vi "save_file_from_netcat.vi"() -> ()   [LabVIEW 2018]
doc: "Demonstrates how to open a connection to an TCP server, read the data being sent, and display the data on a chart. This VI is designed to stop if the TCP connection is terminated."
panel:
  out "bytes received":i32
  out "data":string
  in  "Server Closed":string="The server VI closed the connection."
  in  "Stop":bool
  # "Overview: Demonstrates the use of the TCP functions to connect to a TCP server VI and receive data.\nInstructions:\n1. Ensure Simple TCP - Server.vi is already running.\n2. Run the VI.\n3. Click Stop to stop the VI. Note that if you stop the server VI, this VI will stop automatically."
  # "Send the file on sever using netcat:\nnc -T reliability 192.168.163.61 5901 < OpenSSH-Win64.zip"
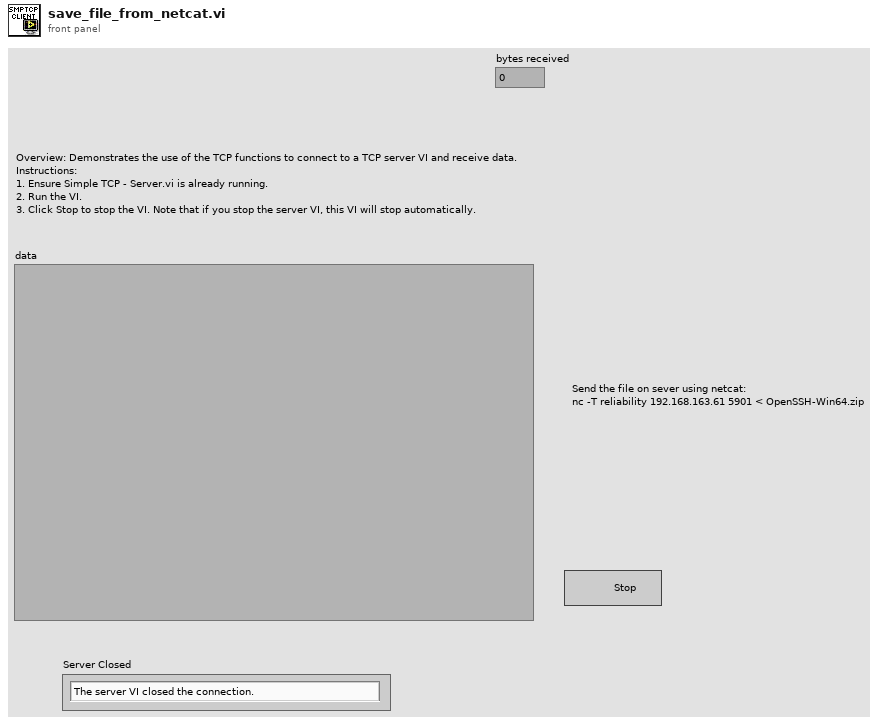
[diagram p1: front panel]
types:
  T1 = enum16{"open", "replace", "create", "open or create", "replace or create", "replace or create with confirmation"}
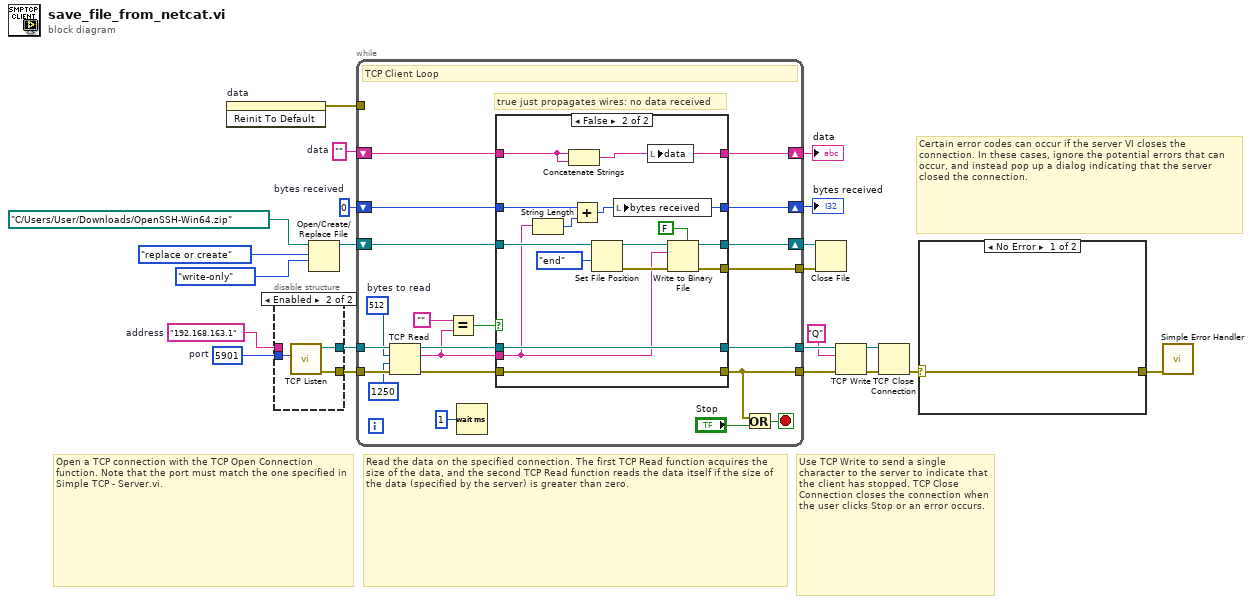
[diagram p0: block diagram]
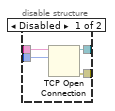
[diagram p2: hidden frame]
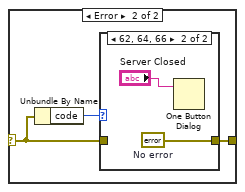
[diagram p3: hidden frame]
diagram:
  w2 = 0  # bytes received
  w11 = ""  # data
  w12 = u16 5901  # port
  w13 = "192.168.163.1"  # address
  # "Certain error codes can occur if the server VI closes the connection. In these cases, ignore the potential errors that can occur, and instead pop up a dialog indicating that the server closed the connection."
  # "Use TCP Write to send a single character to the server to indicate that the client has stopped. TCP Close Connection closes the connection when the user clicks Stop or an error occurs."
  # "Read the data on the specified connection. The first TCP Read function acquires the size of the data, and the second TCP Read function reads the data itself if the size of the data (specified by the server) is greater than zero."
  # "Open a TCP connection with the TCP Open Connection function. Note that the port must match the one specified in Simple TCP - Server.vi."
  n1 = invoke on="data" class="Str" method="Reinit To Default"() -> (error out=w9:errorcluster)  [unwired: 3 in, 2 out]
  n2 = disable-structure shown="Enabled" {
    disable-tunnel: [w26 w28] -> w22
    disable-tunnel: [w25 w29] -> w21
    disable-tunnel: w13 -> [w24 _]
    disable-tunnel: w12 -> [w23 w27]
    frame Disabled {
      n3 = TCP Open Connection(address=w24, remote port or service name=w23) -> (connection ID=w26:refnum<k5>, error out=w25:errorcluster)  [unwired: 3 in]
    }
    frame Enabled {
      n4 = call <vilib>:"TCP Listen.vi"("port"=w27) -> ("error out"=w29:errorcluster, "connection ID"=w28:refnum<k5>)  [unwired: 6 in, 3 out]
    }
  }
  n5 = Open/Create/Replace File(file path (use dialog)=path "C:/Users/User/Downloads/OpenSSH-Win64.zip" ("file (use dialog)"), operation (0:open)=T1."replace or create", access (0:read/write)=enum16{"read/write", "read-only", "write-only"}."write-only") -> (refnum out=w5:refnum<file>)  [unwired: 3 in, 2 out]
  n6 = while {
    tunnel: w21 -> [w47]
    tunnel: w22 -> [w48]
    tunnel: [w43] -> w19
    tunnel: [w42] -> w17
    shift-right: [w40] -> w10
    shift-left: w11 -> [w41]
    tunnel: w9 -> [_]
    tunnel: [w33] -> w4
    shift-right: [w32] -> w3
    shift-left: w5 -> [w34]
    shift-right: [w30] -> w1
    shift-left: w2 -> [w31]
    stop <- w45 stop-if-true
    w39 = 512  # bytes to read
    # "true just propagates wires: no data received"
    # "TCP Client Loop"
    n7 = TCP Read(connection ID=w48, bytes to read=w39, error in (no error)=w47, 9:1250 ("timeout ms (25000)")) -> (connection ID out=w50:refnum<k5>, data out=w35:string, error out=w49:errorcluster)  [unwired: 1 in]
    n8 = Equal?(x="", y=w35) -> (x = y?=w36:bool)
    n9 = Wait (ms)(milliseconds to wait=u32 1) -> ()  [unwired: 1 out]
    n10 = case shown="False" w36 {
      tunnel: w50 -> [w55 w69]
      tunnel: w49 -> [w54 w68]
      tunnel: [w55 w69] -> w43
      tunnel: [w54 w68] -> w42
      tunnel: w41 -> [w53 w60]
      tunnel: [w53 w70] -> w40
      tunnel: w35 -> [_ w59]
      tunnel: w34 -> [w52 w64]
      tunnel: [_ w62] -> w33
      tunnel: [w52 w61] -> w32
      tunnel: w31 -> [w51 w57]
      tunnel: [w51 w56] -> w30
      frame True {
        # "The server has not written any data"
      }
      frame False {
        n11 = String Length(string=w59) -> (length=w58:i32)
        n12 = Concatenate Strings(w60, w60) -> (w70:string)
        n13 = Add(x=w57, y=w58) -> (x+y=w56:i32)
        n14 = Set File Position(refnum=w64, from (0:start)=enum16{"start", "end", "current"}."end") -> (refnum out=w63:refnum<file>, error out=w66:errorcluster)  [unwired: 2 in]
        n15 = local write "bytes received"(w56) -> ()
        n16 = local write "data"(w70) -> ()
        n17 = Write to Binary File(file (use dialog)=w63, data=w59, error in=w66, 5:FALSE ("prepend array or string size? (T)")) -> (refnum out=w61:refnum<file>, error out=w62:errorcluster)  [unwired: 2 in, 1 out]
      }
    }
    n18 = Or(x=w42, y="Stop") -> (x .or. y?=w45:bool)
  }
  "data" <- w10
  "bytes received" <- w1
  n19 = Close File(refnum=w3, error in=w4) -> ()  [unwired: 2 out]
  n20 = TCP Write(connection ID=w19, data in="Q", error in (no error)=w17) -> (connection ID out=w20:refnum<k5>, error out=w18:errorcluster)  [unwired: 2 out]
  n21 = TCP Close Connection(connection ID=w20, error in (no error)=w18) -> (error out=w15:errorcluster)  [unwired: 1 in, 1 out]
  n22 = case shown="No Error" w15 {
    selector: w15 -> [w71 w73]
    tunnel: [w71 w72] -> w14
    frame No Error {
    }
    frame Error {
      n23 = Unbundle By Name(w73) -> ("code"=w74:i32)
      n24 = case shown="62, 64, 66" w74 {
        tunnel: w73 -> [w75 _]
        tunnel: [w75 w77] -> w72
        frame Default {
        }
        frame 62, 64, 66 {
          w77 = errorcluster {"status"=FALSE, "code"=0, "source"=""}  # No error
          n25 = One Button Dialog(message="Server Closed") -> ()  [unwired: 1 in, 1 out]
        }
      }
    }
  }
  n26 = call <vilib>:"Simple Error Handler.vi"("error in (no error)"=w14) -> ()  [unwired: 4 in, 5 out]
